vi "6704_Convert_To_Voltage.vi"(9 "Conversion":T1, 10 "Value":dbl) -> (2 "Voltage":dbl)   [LabVIEW 2015]
uses:
  Controls/6704/static_voltage_conversions.ctl
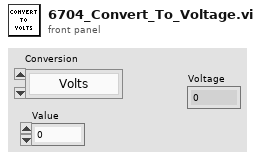
[diagram p1: front panel]
types:
  T1 = typedef "static_voltage_conversions.ctl" = enum16{"Volts", "ODT Power Lock (W)", "Sat Abs Detuning (MHz)", "Blue Mot Power Lock (mW)"}
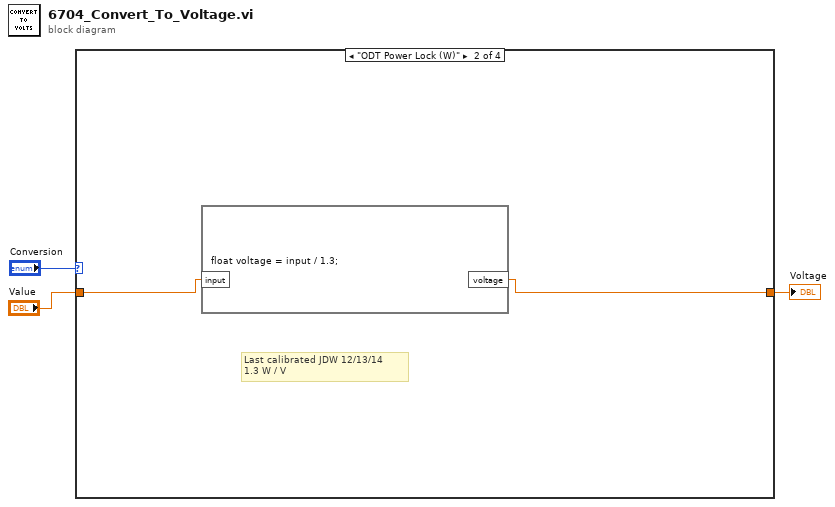
[diagram p0: block diagram]
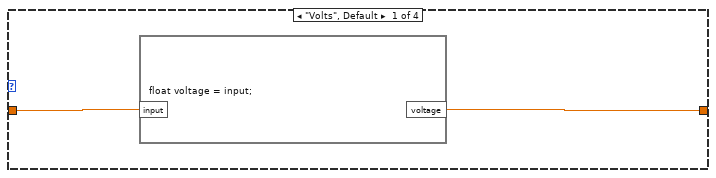
[diagram p2: hidden frame]
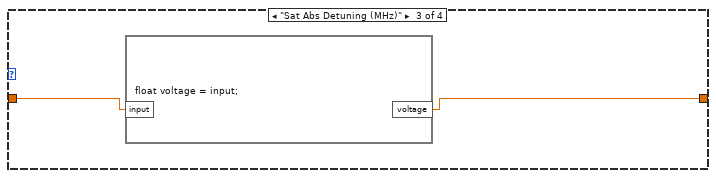
[diagram p3: hidden frame]
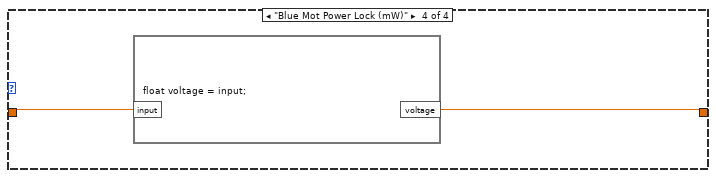
[diagram p4: hidden frame]
diagram:
  n1 = case shown="\"ODT Power Lock (W)\"" "Conversion" {
    tunnel: [w5 w6 w8 w11] -> w2
    tunnel: "Value" -> [w4 w7 w9 w10]
    frame "Volts", Default {
      n2 = formula code="float voltage = input;"("input"=w4) -> ("voltage"=w5:dbl)
    }
    frame "ODT Power Lock (W)" {
      # "Last calibrated JDW 12/13/14\n1.3 W / V"
      n3 = formula code="float voltage = input / 1.3;"("input"=w7) -> ("voltage"=w6:dbl)
    }
    frame "Sat Abs Detuning (MHz)" {
      n4 = formula code="float voltage = input;"("input"=w9) -> ("voltage"=w8:dbl)
    }
    frame "Blue Mot Power Lock (mW)" {
      n5 = formula code="float voltage = input;"("input"=w10) -> ("voltage"=w11:dbl)
    }
  }
  "Voltage" <- w2
